vi "FGV-Module.vi"(6 "Operation":T1(ring), 8 "Error in":errorcluster caption="Error in (no error)", 11 "input":dbl) -> (0 "Error out":errorcluster, 3 "dbl":dbl)   [LabVIEW 2020]
uses:
  DataDef.ctl
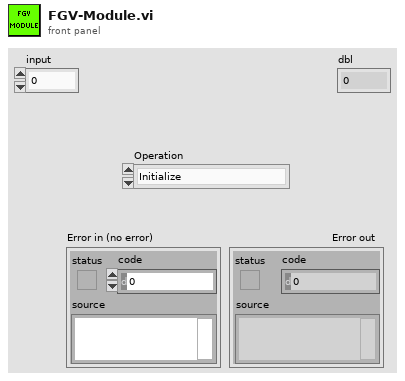
[diagram p1: front panel]
types:
  T1 = enum16{"Initialize", "Random", "Read", "Write", "Close"}
  T2 = typedef "DataDef.ctl" = cluster{"dbl":dbl}
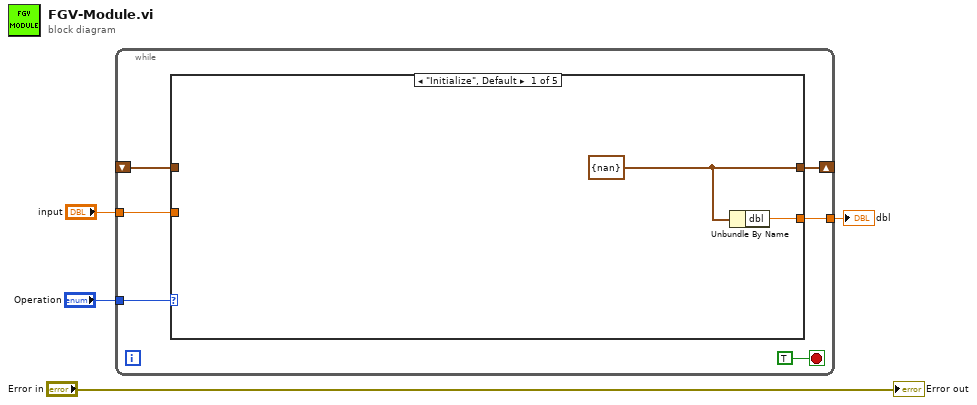
[diagram p0: block diagram]
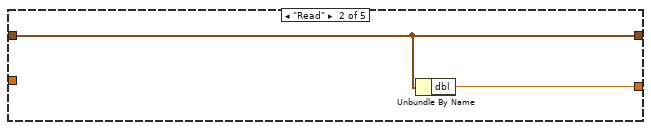
[diagram p2: hidden frame]
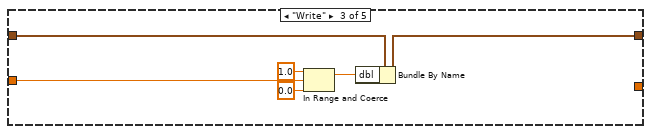
[diagram p3: hidden frame]
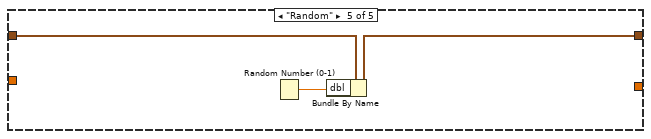
[diagram p5: hidden frame]
diagram:
  n1 = while {
    tunnel: "Operation" -> [w9]
    shift-right: [w8] -> _
    shift-left: _ -> [w7]
    tunnel: [w6] -> w3
    tunnel: "input" -> [w5]
    stop <- TRUE stop-if-true
    n2 = case shown="\"Initialize\", Default" w9 {
      tunnel: [w11 w14 w19 _ w22] -> w8
      tunnel: w7 -> [_ w14 w20 _ w23]
      tunnel: [w12 w13 _ _ _] -> w6
      tunnel: w5 -> [_ _ w17 _ _]
      frame "Initialize", Default {
        w11 = T2 {"dbl"=nan} ("ModuleData")
        n3 = Unbundle By Name(w11) -> ("dbl"=w12:dbl)
      }
      frame "Read" {
        n4 = Unbundle By Name(w14) -> ("dbl"=w13:dbl)
      }
      frame "Write" {
        n5 = In Range and Coerce(upper limit=1.0, x=w17, lower limit=0.0) -> (coerced(x)=w18:dbl)  [unwired: 1 out]
        n6 = Bundle By Name(cluster=w20, "dbl"=w18) -> (w19:T2)
      }
      frame "Close" {
      }
      frame "Random" {
        n7 = Random Number (0-1)() -> (number: 0 to 1=w21:dbl)
        n8 = Bundle By Name(cluster=w23, "dbl"=w21) -> (w22:T2)
      }
    }
  }
  "dbl" <- w3
  "Error out" <- "Error in"
